vi "ShiftRegister FeedbackNode Difference.vi"() -> ()   [LabVIEW 2014]
panel:
  out "FeedbackNode array":string[](array[string])
  out "ShiftRegister array":string[](array[string])
  # "These array should be different, that what I was thinking, but they are same, probably my mistake :(\nBut I learn it now."
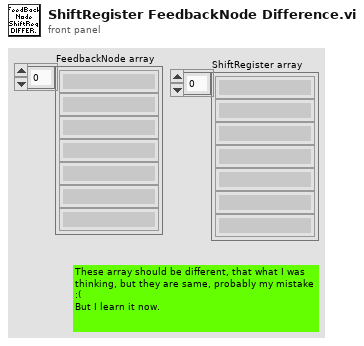
[diagram p1: front panel]
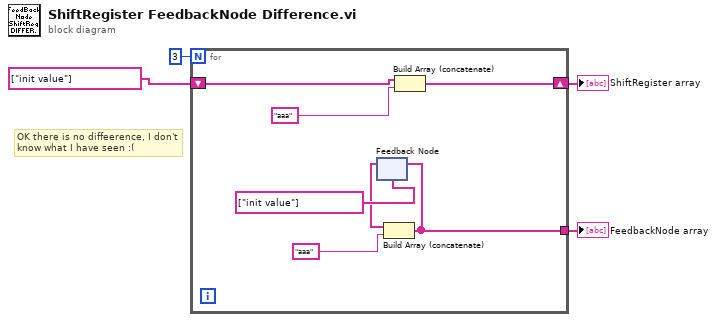
[diagram p0: block diagram]
diagram:
  # "OK there is no diffeerence, I don't\nknow what I have seen :("
  n1 = for {
    N: 3 -> [_]
    shift-right: [w10] -> w3
    shift-left: string[] ["init value"] -> [w11]
    tunnel: [w5] -> w1
    n2 = feedback #1(string[] ["init value"]) -> (w6:string[])
    n3 = Build Array (concatenate)(w6, "aaa") -> (w5:string[])
    n4 = feedback-in #1(w5) -> ()
    n5 = Build Array (concatenate)(w11, "aaa") -> (w10:string[])
  }
  "ShiftRegister array" <- w3
  "FeedbackNode array" <- w1
